vi "PRax12.3.3.vi"   [LabVIEW 2020]
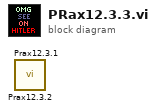
[diagram p0: block diagram]
diagram:
  n1 = call "Prax12.3.2.vi"() -> ()  [unwired: 11 in, 1 out]
  n2 = call "Prax12.3.1.vi"() -> ()  [unwired: 11 in, 1 out]
